vi "Dashboard Receive Packet.vi"(11 "connection ID":refnum<k16>) -> ()   [LabVIEW 2017]
uses:
  Common Code/Dashboard Control Data.ctl
  Common Code/Drivetrain Settings Clustr.ctl
  Common Code/PID Gains Cluster.ctl
  Common Code/Encoder Values.ctl
  Common Code/Intake Presets.ctl
  Common Code/Elevator Settings Cluster.ctl
  Common Code/PID Gains.ctl
  Robot Global Data.vi
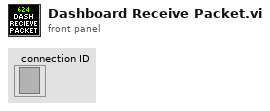
[diagram p1: front panel]
types:
  T1 = typedef "Dashboard Control Data.ctl" = cluster{"Drivetrain Settings Cluster":T2, "Intake Presets":T5, "Elevator Settings Cluster":T6}
  T2 = typedef "Drivetrain Settings Clustr.ctl" = cluster{"Gyro Steer PID Gains":T3, "Distance Drive PID Gains":T3, "Encoder Values":T4, "Drive Tolerance":dbl, "Gyro Tolerance":dbl, "Gyro Output":dbl, "Distance Output":dbl, "Y Power Multiplier":dbl, "Turn Power Multiplier":dbl, "Creep Rate":dbl, "Constant Power":bool, "DT Input Modifier":enum16{"None", "Cube", "Square"}}
  T3 = typedef "PID Gains Cluster.ctl" = cluster{"Integral Time":dbl, "Proportional Gain":dbl, "Derivative Time":dbl}
  T4 = typedef "Encoder Values.ctl" = cluster{"Left Encoder Values":cluster{"Distance":dbl, "Speed":dbl, "Tick":dbl}, "Right Encoder Values":cluster{"Distance":dbl, "Speed":dbl, "Tick":dbl}}
  T5 = typedef "Intake Presets.ctl" = cluster{"Idle Angle":dbl, "Mid Angle":dbl, "Low Angle":dbl, "Outtake Power":dbl, "Intake Power":dbl, "Unstuck":dbl, "Angle Tolerance":dbl, "Max Angle":dbl, "Max Current":dbl, "Current Trip Time":dbl, "Reset Encoder?":bool, "Encoder Scale":dbl, "PID gains":cluster{"proportional gain (Kc)":dbl, "integral time (Ti, min)":dbl, "derivative time (Td, min)":dbl}, "output range":cluster{"output high":dbl, "output low":dbl}}
  T6 = typedef "Elevator Settings Cluster.ctl" = cluster{"Ground Height":dbl, "Switch Height":dbl, "Scale High Height ":dbl, "Scale Low Height":dbl, "Elevator PID Gains":T7, "Elevator Tolerance":dbl, "Reset Encoders":bool, "Encoder Scale":dbl, "Max Height":dbl, "Mid Height":dbl, "output range":cluster{"output high":dbl, "output low":dbl}}
  T7 = typedef "PID Gains.ctl" = cluster{"proportional gain (Kc)":dbl, "integral time (Ti, min)":dbl, "derivative time (Td, min)":dbl}
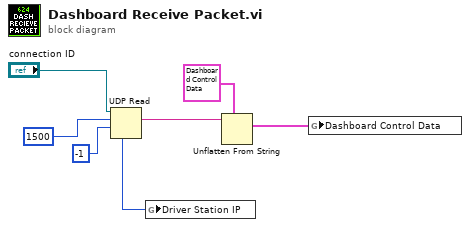
[diagram p0: block diagram]
diagram:
  n1 = UDP Read(connection ID="connection ID", max size (548)=1500, timeout ms (25000)=-1) -> (data out=w5:string, 6:w2:u32)  [unwired: 1 in, 3 out]
  n2 = global write "Robot Global Data.vi" "Driver Station IP"(w2) -> ()
  n3 = Unflatten From String(type=T1 {"Drivetrain Settings Cluster"={"Gyro Steer PID Gains"={"Integral Time"=0.0, "Proportional Gain"=0.0, "Derivative Time"=0.0}, "Distance Drive PID Gains"={"Integral Time"=0.0, "Proportional Gain"=0.0, "Derivative Time"=0.0}, "Encoder Values"={"Left Encoder Values"={"Distance"=0.0, "Speed"=0.0, "Tick"=0.0}, "Right Encoder Values"={"Distance"=0.0, "Speed"=0.0, "Tick"=0.0}}, "Drive Tolerance"=0.0, "Gyro Tolerance"=0.0, "Gyro Output"=0.0, "Distance Output"=0.0, "Y Power Multiplier"=0.0, "Turn Power Multiplier"=0.0, "Creep Rate"=0.0, "Constant Power"=FALSE, "DT Input Modifier"=enum."None"}, "Intake Presets"={"Idle Angle"=0.0, "Mid Angle"=0.0, "Low Angle"=0.0, "Outtake Power"=0.0, "Intake Power"=0.0, "Unstuck"=0.0, "Angle Tolerance"=0.0, "Max Angle"=0.0, "Max Current"=0.0, "Current Trip Time"=0.0, "Reset Encoder?"=FALSE, "Encoder Scale"=0.0, "PID gains"={"proportional gain (Kc)"=0.0, "integral time (Ti, min)"=0.0, "derivative time (Td, min)"=0.0}, "output range"={"output high"=100.0, "output low"=-100.0}}, "Elevator Settings Cluster"={"Ground Height"=0.0, "Switch Height"=0.0, "Scale High Height "=0.0, "Scale Low Height"=0.0, "Elevator PID Gains"={"proportional gain (Kc)"=1.0, "integral time (Ti, min)"=0.01, "derivative time (Td, min)"=0.0}, "Elevator Tolerance"=0.0, "Reset Encoders"=FALSE, "Encoder Scale"=0.0, "Max Height"=0.0, "Mid Height"=0.0, "output range"={"output high"=0.0, "output low"=0.0}}} ("Dashboard Control Data"), binary string=w5) -> (value=w1:T1)  [unwired: 3 in, 2 out]
  n4 = global write "Robot Global Data.vi" "Dashboard Control Data"(w1) -> ()
